vi "FeedbackDecode_20200902.vi"() -> ()   [LabVIEW 2016] (continued)
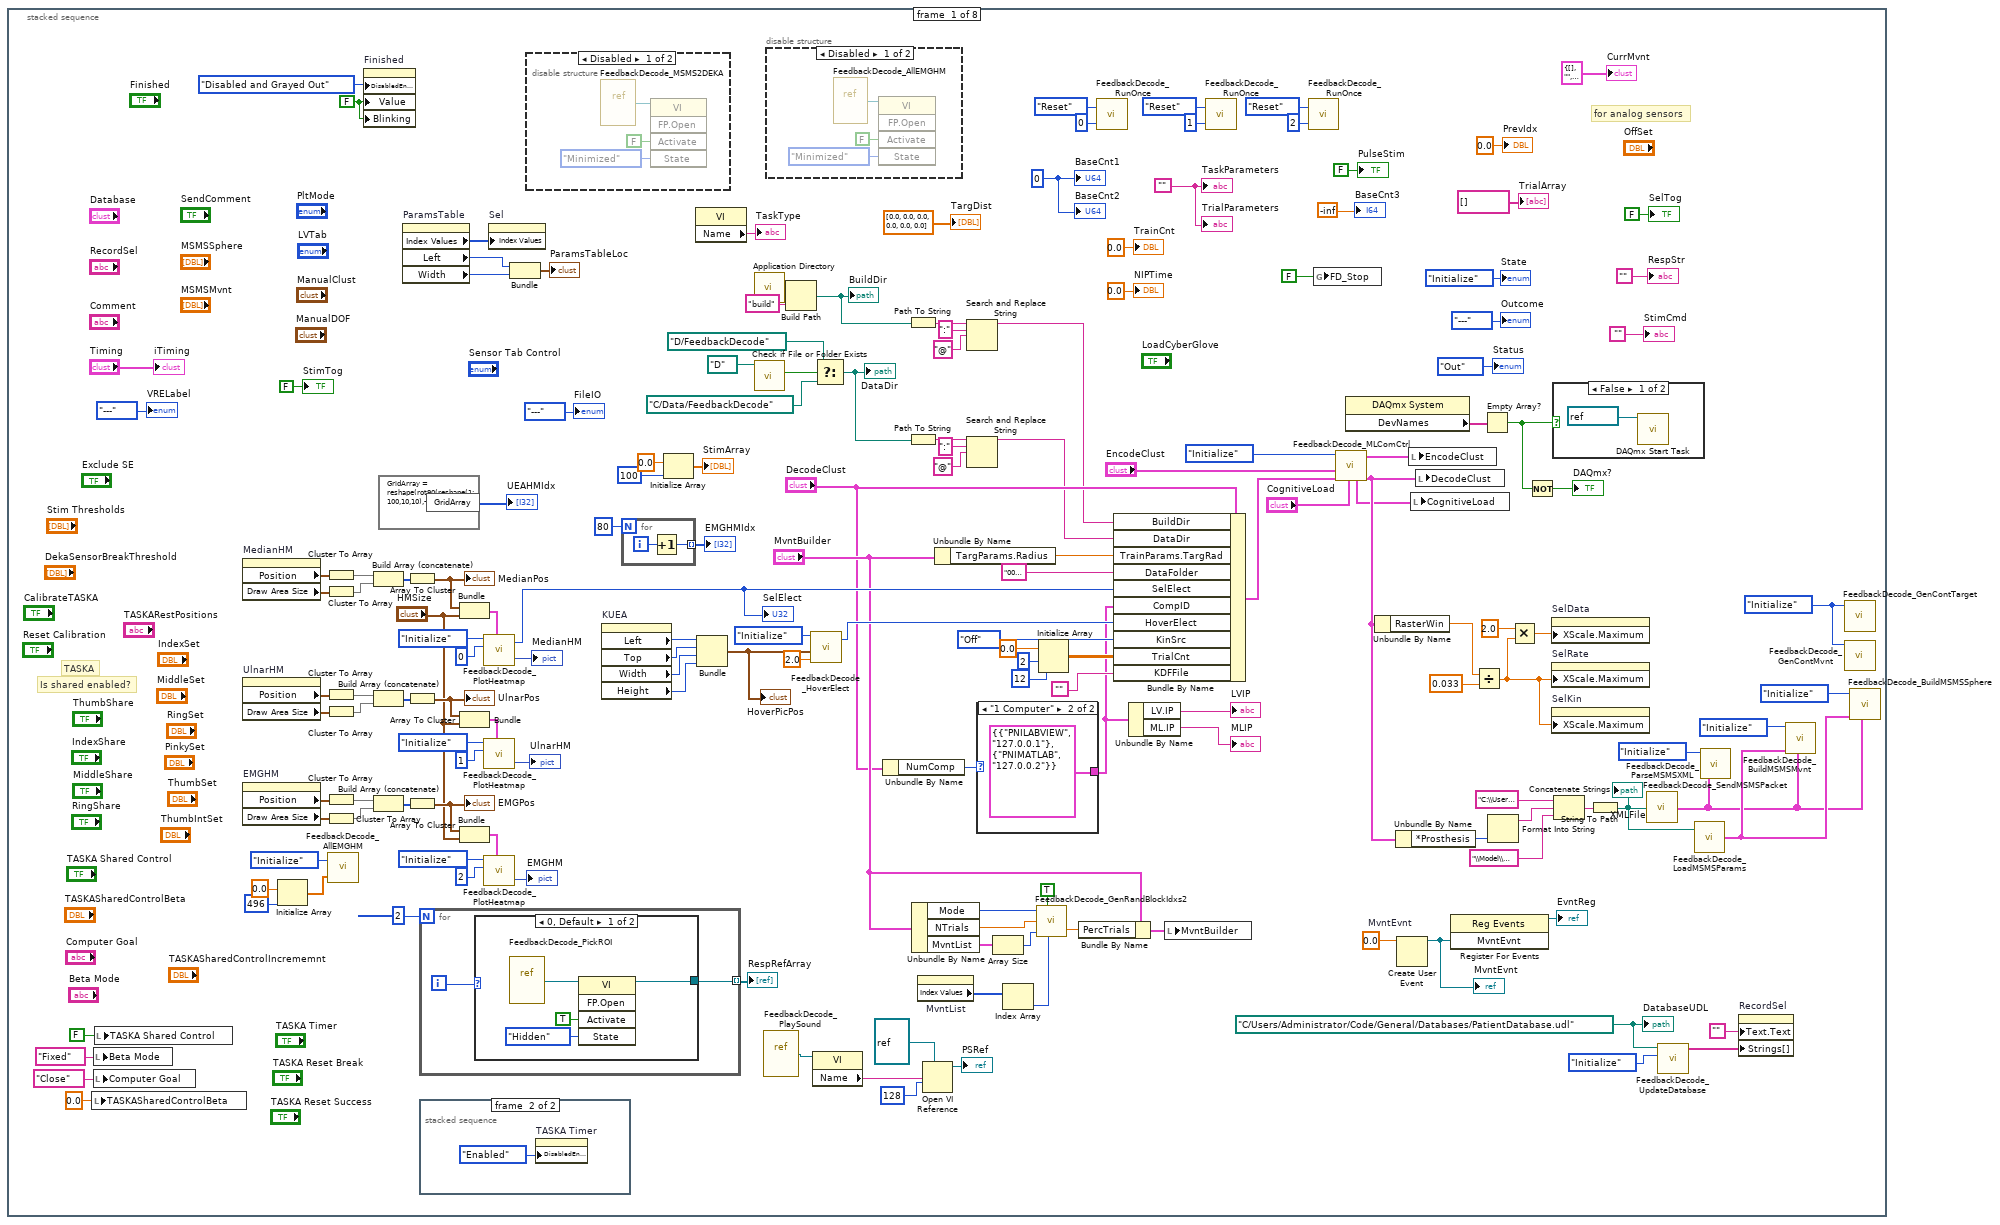
[diagram p2: hidden frame]
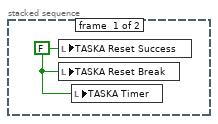
[diagram p3: hidden frame]
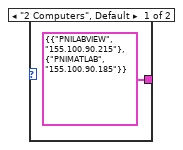
[diagram p4: hidden frame]
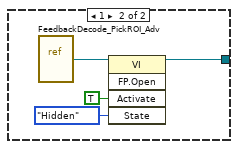
[diagram p7: hidden frame]
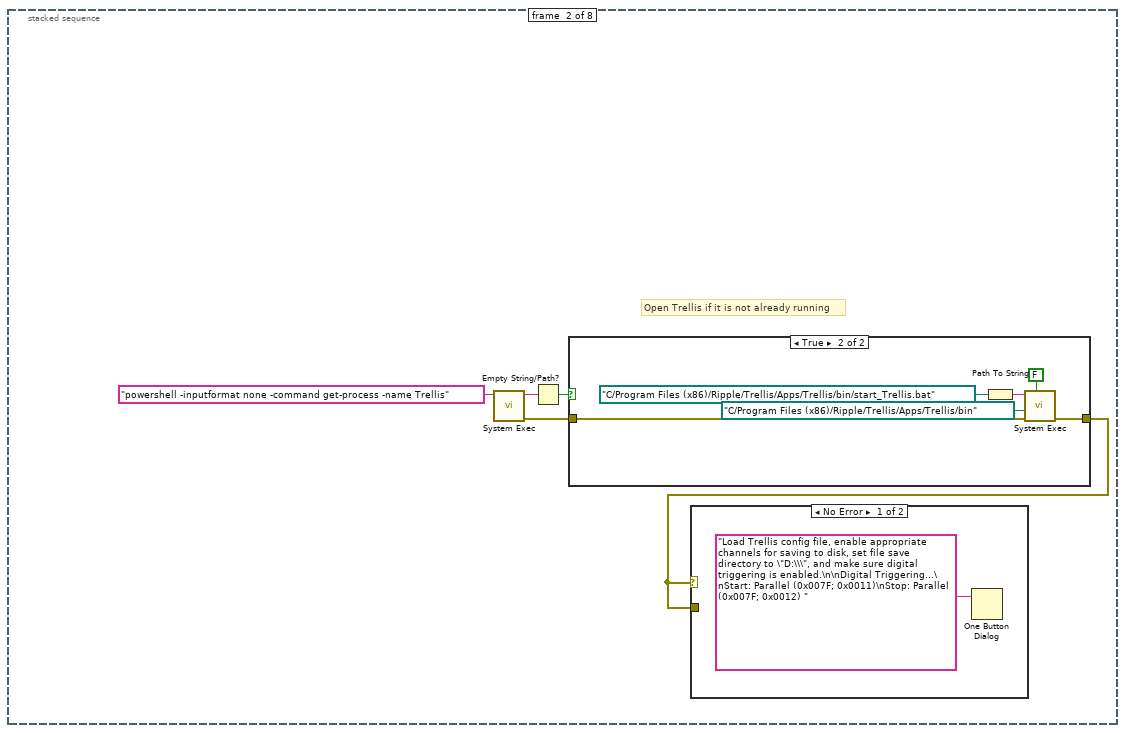
[diagram p9: hidden frame]
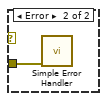
[diagram p11: hidden frame]
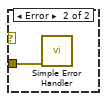
[diagram p14: hidden frame]
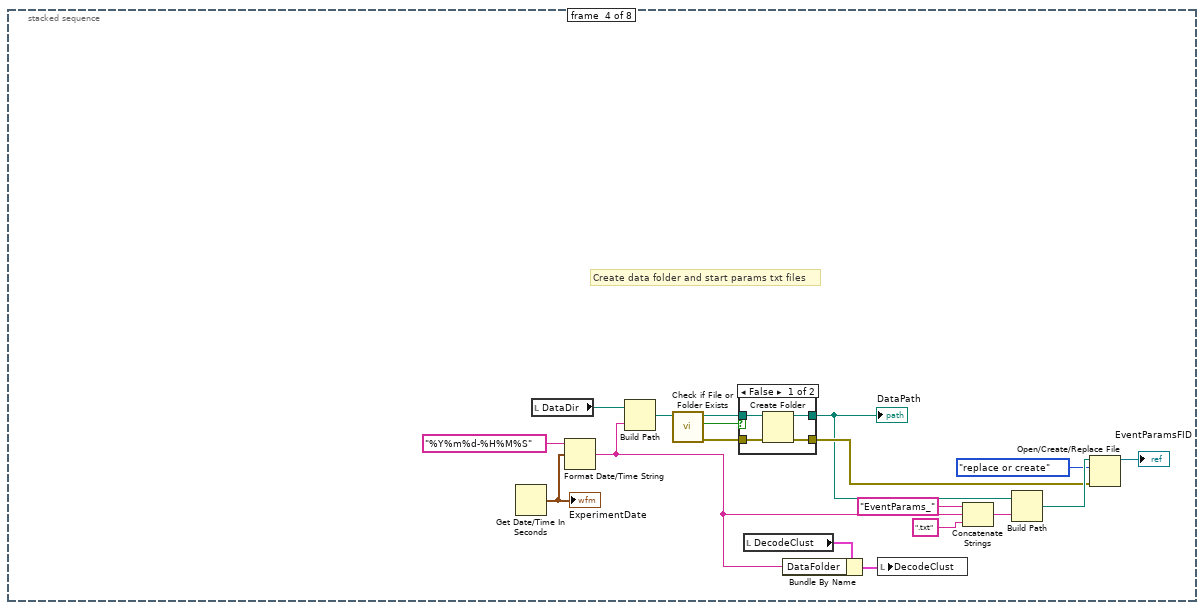
[diagram p15: hidden frame]
              }
              frame False {
                n2368 = property on="TASKA Timer" class="Bool (strict)"("DisabledEnum"=T17."Disabled and Grayed Out" ("Disabled")) -> ()  [unwired: 2 in, 2 out]
                n2369 = local read "LoopCnt"() -> (w2592:u64)
                n2370 = local read "NIPTime"() -> (w2595:dbl)
                n2371 = Format Into String(w2592) -> (resulting string=w2599:string)  [unwired: 3 in, 1 out]
                n2372 = local read "EventParamsFID"() -> (w2589:refnum<file>)
                n2373 = Concatenate Strings("SharedControlStopTime:SS.EventID=" ("string"), w2599) -> (w2593:string)
                n2374 = call-poly "FeedbackDecode_VariablesToString.vi"("Format"="%0.0f", "ValueIn"=w2595, "FieldName"="NIPTime" ("Key Word")) -> ("StringOut"=w2598:string)  [unwired: 4 in]
                n2375 = Concatenate Strings(w2593, ";", w2598) -> (w2594:string)
                n2376 = call "FeedbackDecode_WriteTextEOL.vi"("text"=w2594, "refnum in"=w2589) -> ()  [unwired: 8 in, 2 out]
              }
            }
          }
          event "TASKA Reset Break": Value Change {
            n2377 = event-data() -> ()  [unwired: 1 in, 6 out]
            n2378 = call-poly "FeedbackDecode_VariablesToString.vi"("Format"="%0.0f", "ValueIn"=0.0, "FieldName"="SharedControlTrialSuccess" ("Key Word")) -> ("StringOut"=w2601:string)  [unwired: 4 in]
            n2379 = property on="TASKA Timer" class="Bool (strict)"("DisabledEnum"=T17."Enabled" ("Disabled")) -> ()  [unwired: 2 in, 2 out]
            n2380 = local read "LoopCnt"() -> (w2608:u64)
            n2381 = local read "NIPTime"() -> (w2611:dbl)
            n2382 = Format Into String(w2608) -> (resulting string=w2615:string)  [unwired: 3 in, 1 out]
            n2383 = local read "EventParamsFID"() -> (w2605:refnum<file>)
            n2384 = Concatenate Strings("SharedControlTrialResult:SS.EventID=" ("string"), w2615) -> (w2609:string)
            n2385 = call-poly "FeedbackDecode_VariablesToString.vi"("Format"="%0.0f", "ValueIn"=w2611, "FieldName"="NIPTime" ("Key Word")) -> ("StringOut"=w2614:string)  [unwired: 4 in]
            n2386 = Concatenate Strings(w2609, ";", w2601, w2614) -> (w2610:string)
            n2387 = call "FeedbackDecode_WriteTextEOL.vi"("text"=w2610, "refnum in"=w2605) -> ()  [unwired: 8 in, 2 out]
          }
          event "TASKA Reset Success": Value Change {
            n2388 = event-data() -> ()  [unwired: 1 in, 6 out]
            n2389 = call-poly "FeedbackDecode_VariablesToString.vi"("Format"="%0.0f", "ValueIn"=1.0, "FieldName"="SharedControlTrialSuccess" ("Key Word")) -> ("StringOut"=w2618:string)  [unwired: 4 in]
            n2390 = property on="TASKA Timer" class="Bool (strict)"("DisabledEnum"=T17."Enabled" ("Disabled")) -> ()  [unwired: 2 in, 2 out]
            n2391 = local read "LoopCnt"() -> (w2625:u64)
            n2392 = local read "NIPTime"() -> (w2628:dbl)
            n2393 = Format Into String(w2625) -> (resulting string=w2632:string)  [unwired: 3 in, 1 out]
            n2394 = local read "EventParamsFID"() -> (w2622:refnum<file>)
            n2395 = Concatenate Strings("SharedControlTrialResult:SS.EventID=" ("string"), w2632) -> (w2626:string)
            n2396 = call-poly "FeedbackDecode_VariablesToString.vi"("Format"="%0.0f", "ValueIn"=w2628, "FieldName"="NIPTime" ("Key Word")) -> ("StringOut"=w2631:string)  [unwired: 4 in]
            n2397 = Concatenate Strings(w2626, ";", w2618, w2631) -> (w2627:string)
            n2398 = call "FeedbackDecode_WriteTextEOL.vi"("text"=w2627, "refnum in"=w2622) -> ()  [unwired: 8 in, 2 out]
          }
          event "TASKASharedControlBeta": Value Change {
            n2399 = event-data() -> ("NewVal"=w2634:dbl)  [unwired: 1 in, 5 out]
            n2400 = local read "LoopCnt"() -> (w2644:u64)
            n2401 = call-poly "FeedbackDecode_VariablesToString.vi"("Format"="%0.5f", "ValueIn"=w2634, "FieldName"="TASKASensors.SharedControl.Beta") -> ("StringOut"=w2651:string)  [unwired: 4 in]
            n2402 = local read "NIPTime"() -> (w2640:dbl)
            n2403 = Format Into String(w2644) -> (resulting string=w2636:string)  [unwired: 3 in, 1 out]
            n2404 = local read "EventParamsFID"() -> (w2648:refnum<file>)
            n2405 = local read "DecodeClust"() -> (w2649:T5)
            n2406 = Concatenate Strings("SharedControl:SS.EventID=" ("string"), w2636) -> (w2643:string)
            n2407 = call-poly "FeedbackDecode_VariablesToString.vi"("Format"="%0.0f", "ValueIn"=w2640, "FieldName"="NIPTime" ("Key Word")) -> ("StringOut"=w2637:string)  [unwired: 4 in]
            n2408 = Concatenate Strings(w2643, ";", w2651, w2637) -> (w2642:string)
            n2409 = call "FeedbackDecode_WriteTextEOL.vi"("text"=w2642, "refnum in"=w2648) -> ()  [unwired: 8 in, 2 out]
            n2410 = Bundle By Name(cluster=w2649, "EventStr"=w2642) -> (w2641:T5)
            n2411 = call "FeedbackDecode_MLComCtrl.vi"("DecodeClustIn"=w2641, "Mode"=T19."SendEvent") -> ()  [unwired: 6 in, 4 out]
          }
          event "TASKASharedControlIncrememnt": Value Change {
            n2412 = event-data() -> ("NewVal"=w2653:dbl)  [unwired: 1 in, 5 out]
            n2413 = local read "LoopCnt"() -> (w2663:u64)
            n2414 = call-poly "FeedbackDecode_VariablesToString.vi"("Format"="%0.5f", "ValueIn"=w2653, "FieldName"="TASKASensors.SharedControl.Increment") -> ("StringOut"=w2670:string)  [unwired: 4 in]
            n2415 = local read "NIPTime"() -> (w2659:dbl)
            n2416 = Format Into String(w2663) -> (resulting string=w2655:string)  [unwired: 3 in, 1 out]
            n2417 = local read "EventParamsFID"() -> (w2667:refnum<file>)
            n2418 = local read "DecodeClust"() -> (w2668:T5)
            n2419 = Concatenate Strings("SharedControl:SS.EventID=" ("string"), w2655) -> (w2662:string)
            n2420 = call-poly "FeedbackDecode_VariablesToString.vi"("Format"="%0.0f", "ValueIn"=w2659, "FieldName"="NIPTime" ("Key Word")) -> ("StringOut"=w2656:string)  [unwired: 4 in]
            n2421 = Concatenate Strings(w2662, ";", w2670, w2656) -> (w2661:string)
            n2422 = call "FeedbackDecode_WriteTextEOL.vi"("text"=w2661, "refnum in"=w2667) -> ()  [unwired: 8 in, 2 out]
            n2423 = Bundle By Name(cluster=w2668, "EventStr"=w2661) -> (w2660:T5)
            n2424 = call "FeedbackDecode_MLComCtrl.vi"("DecodeClustIn"=w2660, "Mode"=T19."SendEvent") -> ()  [unwired: 6 in, 4 out]
          }
          event "IndexSet", "MiddleSet", "RingSet", "PinkySet", "ThumbSet", "ThumbIntSet": Value Change {
            n2425 = event-data() -> ()  [unwired: 1 in, 6 out]
            n2426 = local read "ThumbIntSet"() -> (w2672:dbl)
            n2427 = local read "ThumbSet"() -> (w2673:dbl)
            n2428 = local read "MiddleSet"() -> (w2678:dbl)
            n2429 = local read "RingSet"() -> (w2677:dbl)
            n2430 = local read "PinkySet"() -> (w2674:dbl)
            n2431 = local read "IndexSet"() -> (w2679:dbl)
            n2432 = Build Array(w2679, w2678, w2677, w2674, w2673, w2672) -> (w2676:dbl[])
            n2433 = local read "LoopCnt"() -> (w2688:u64)
            n2434 = call-poly "FeedbackDecode_VariablesToString.vi"("Format"="%0.5f", "ValueIn"=w2676, "FieldName"="TASKA.RestPositions") -> ("StringOut"=w2695:string)  [unwired: 4 in]
            n2435 = local read "NIPTime"() -> (w2684:dbl)
            n2436 = Format Into String(w2688) -> (resulting string=w2681:string)  [unwired: 3 in, 1 out]
            n2437 = local read "EventParamsFID"() -> (w2692:refnum<file>)
            n2438 = local read "DecodeClust"() -> (w2693:T5)
            n2439 = Concatenate Strings("SharedControl:SS.EventID=" ("string"), w2681) -> (w2687:string)
            n2440 = call-poly "FeedbackDecode_VariablesToString.vi"("Format"="%0.0f", "ValueIn"=w2684, "FieldName"="NIPTime" ("Key Word")) -> ("StringOut"=w2675:string)  [unwired: 4 in]
            n2441 = Concatenate Strings(w2687, ";", w2695, w2675) -> (w2686:string)
            n2442 = call "FeedbackDecode_WriteTextEOL.vi"("text"=w2686, "refnum in"=w2692) -> ()  [unwired: 8 in, 2 out]
            n2443 = Bundle By Name(cluster=w2693, "EventStr"=w2686) -> (w2685:T5)
            n2444 = call "FeedbackDecode_MLComCtrl.vi"("DecodeClustIn"=w2685, "Mode"=T19."SendEvent") -> ()  [unwired: 6 in, 4 out]
          }
          event "ThumbShare", "IndexShare", "MiddleShare", "RingShare": Value Change {
            n2445 = event-data() -> ()  [unwired: 1 in, 6 out]
            n2446 = local read "ThumbShare"() -> (w2700:bool)
            n2447 = local read "MiddleShare"() -> (w2704:bool)
            n2448 = local read "RingShare"() -> (w2703:bool)
            n2449 = local read "IndexShare"() -> (w2705:bool)
            n2450 = Build Array(w2705, w2704, w2703, FALSE ("element"), w2700, FALSE ("element")) -> (w2698:bool[])
            n2451 = for {
              tunnel: w2698 -> [w2724] mode=indexing
              tunnel: [w2723] -> w2697 mode=indexing
              n2452 = case shown="False" w2724 {
                tunnel: [0.0 ("ValueIn") 1.0 ("ValueIn")] -> w2723
                frame False {
                }
                frame True {
                }
              }
            }
            n2453 = local read "LoopCnt"() -> (w2714:u64)
            n2454 = local read "NIPTime"() -> (w2710:dbl)
            n2455 = call-poly "FeedbackDecode_VariablesToString.vi"("Format"="%1.0f", "ValueIn"=w2697, "FieldName"="TASKASensors.SharedEnabled") -> ("StringOut"=w2721:string)  [unwired: 4 in]
            n2456 = Format Into String(w2714) -> (resulting string=w2707:string)  [unwired: 3 in, 1 out]
            n2457 = local read "EventParamsFID"() -> (w2718:refnum<file>)
            n2458 = local read "DecodeClust"() -> (w2719:T5)
            n2459 = Concatenate Strings("SharedControl:SS.EventID=" ("string"), w2707) -> (w2713:string)
            n2460 = call-poly "FeedbackDecode_VariablesToString.vi"("Format"="%0.0f", "ValueIn"=w2710, "FieldName"="NIPTime" ("Key Word")) -> ("StringOut"=w2702:string)  [unwired: 4 in]
            n2461 = Concatenate Strings(w2713, ";", w2721, w2702) -> (w2712:string)
            n2462 = call "FeedbackDecode_WriteTextEOL.vi"("text"=w2712, "refnum in"=w2718) -> ()  [unwired: 8 in, 2 out]
            n2463 = Bundle By Name(cluster=w2719, "EventStr"=w2712) -> (w2711:T5)
            n2464 = call "FeedbackDecode_MLComCtrl.vi"("DecodeClustIn"=w2711, "Mode"=T19."SendEvent") -> ()  [unwired: 6 in, 4 out]
          }
          event "Computer Goal": Value Change {
            n2465 = event-data() -> ("NewVal"=w2727:string)  [unwired: 1 in, 5 out]
            n2466 = local read "LoopCnt"() -> (w2737:u64)
            n2467 = call-poly "FeedbackDecode_VariablesToString.vi"("Format"="%0.5f", "ValueIn"=w2727, "FieldName"="TASKASensors.SharedControl.ComputerGoal") -> ("StringOut"=w2744:string)  [unwired: 4 in]
            n2468 = local read "NIPTime"() -> (w2733:dbl)
            n2469 = Format Into String(w2737) -> (resulting string=w2729:string)  [unwired: 3 in, 1 out]
            n2470 = local read "EventParamsFID"() -> (w2741:refnum<file>)
            n2471 = local read "DecodeClust"() -> (w2742:T5)
            n2472 = Concatenate Strings("SharedControl:SS.EventID=" ("string"), w2729) -> (w2736:string)
            n2473 = call-poly "FeedbackDecode_VariablesToString.vi"("Format"="%0.0f", "ValueIn"=w2733, "FieldName"="NIPTime" ("Key Word")) -> ("StringOut"=w2730:string)  [unwired: 4 in]
            n2474 = Concatenate Strings(w2736, ";", w2744, w2730) -> (w2735:string)
            n2475 = call "FeedbackDecode_WriteTextEOL.vi"("text"=w2735, "refnum in"=w2741) -> ()  [unwired: 8 in, 2 out]
            n2476 = Bundle By Name(cluster=w2742, "EventStr"=w2735) -> (w2734:T5)
            n2477 = call "FeedbackDecode_MLComCtrl.vi"("DecodeClustIn"=w2734, "Mode"=T19."SendEvent") -> ()  [unwired: 6 in, 4 out]
          }
          event "Beta Mode": Value Change {
            n2478 = event-data() -> ("NewVal"=w2746:string)  [unwired: 1 in, 5 out]
            n2479 = local read "LoopCnt"() -> (w2756:u64)
            n2480 = call-poly "FeedbackDecode_VariablesToString.vi"("Format"="%0.5f", "ValueIn"=w2746, "FieldName"="TASKASensors.SharedControl.BetaMode") -> ("StringOut"=w2763:string)  [unwired: 4 in]
            n2481 = local read "NIPTime"() -> (w2752:dbl)
            n2482 = Format Into String(w2756) -> (resulting string=w2748:string)  [unwired: 3 in, 1 out]
            n2483 = local read "EventParamsFID"() -> (w2760:refnum<file>)
            n2484 = local read "DecodeClust"() -> (w2761:T5)
            n2485 = Concatenate Strings("SharedControl:SS.EventID=" ("string"), w2748) -> (w2755:string)
            n2486 = call-poly "FeedbackDecode_VariablesToString.vi"("Format"="%0.0f", "ValueIn"=w2752, "FieldName"="NIPTime" ("Key Word")) -> ("StringOut"=w2749:string)  [unwired: 4 in]
            n2487 = Concatenate Strings(w2755, ";", w2763, w2749) -> (w2754:string)
            n2488 = call "FeedbackDecode_WriteTextEOL.vi"("text"=w2754, "refnum in"=w2760) -> ()  [unwired: 8 in, 2 out]
            n2489 = Bundle By Name(cluster=w2761, "EventStr"=w2754) -> (w2753:T5)
            n2490 = call "FeedbackDecode_MLComCtrl.vi"("DecodeClustIn"=w2753, "Mode"=T19."SendEvent") -> ()  [unwired: 6 in, 4 out]
          }
          event Mouse Wheel; Mouse Down; Mouse Move {
            n2491 = event-data() -> ("CtlRef"=w2765:refnum<vi>)  [unwired: 1 in, 4 out]
            n2492 = property class="Arr (strict)"(reference=w2765) -> ("Index Values"=w2766:u32[])  [unwired: 1 in, 2 out]
            n2493 = Index Array(array=w2766) -> (element=w2767:u32)  [unwired: 1 in]
            n2494 = Build Array(w2767) -> (w2768:u32[])
            n2495 = property on="Sel" class="Arr (strict)"("Index Values"=w2768) -> ()  [unwired: 2 in, 2 out]
          }
          event "RespStr": Value Change {
            n2496 = event-data() -> ("NewVal"=w2770:string)  [unwired: 1 in, 5 out]
            n2497 = Empty String/Path?(string/path=w2770) -> (empty?=w2771:bool)
            n2498 = case shown="False" w2771 {
              tunnel: w2770 -> [w2775 _]
              frame False {
                n2499 = xnode "Match Regular Expression"("input string"=w2775, "regular expression"="Sensor='") -> ("after match"=w2778:string)  [unwired: 4 in, 4 out]
                n2500 = local read "EncodeClust"() -> (w2780:T9)
                n2501 = xnode "Match Regular Expression"("input string"=w2778, "regular expression"="';") -> ("before match"=w2774:string)  [unwired: 4 in, 4 out]
                n2502 = call "FeedbackDecode_UpdateRegion.vi"("EncodeClustIn"=w2780, "RegionStr"=w2774) -> ("EncodeClustOut"=w2779:T9)  [unwired: 1 in]
                n2503 = local write "EncodeClust"(w2779) -> ()
                n2504 = local read "LoopCnt"() -> (w2790:u64)
                n2505 = local read "NIPTime"() -> (w2786:dbl)
                n2506 = local read "StimCmd"() -> (w2773:string)
                n2507 = Format Into String(w2790) -> (resulting string=w2781:string)  [unwired: 3 in, 1 out]
                n2508 = call-poly "FeedbackDecode_VariablesToString.vi"("Format"="%0.0f", "ValueIn"=w2786, "FieldName"="NIPTime" ("Key Word")) -> ("StringOut"=w2783:string)  [unwired: 4 in]
                n2509 = Concatenate Strings("Response:SS.EventID=" ("string"), w2781) -> (w2789:string)
                n2510 = local read "EventParamsFID"() -> (w2793:refnum<file>)
                n2511 = Concatenate Strings(w2789, ";", w2775, w2773, w2783) -> (w2788:string)
                n2512 = local read "DecodeClust"() -> (w2794:T5)
                n2513 = call "FeedbackDecode_WriteTextEOL.vi"("text"=w2788, "refnum in"=w2793) -> ()  [unwired: 8 in, 2 out]
                n2514 = Bundle By Name(cluster=w2794, "EventStr"=w2788) -> (w2787:T5)
                n2515 = call "FeedbackDecode_MLComCtrl.vi"("DecodeClustIn"=w2787, "Mode"=T19."SendEvent") -> ()  [unwired: 6 in, 4 out]
              }
              frame True {
              }
            }
          }
          event Value Change {
            n2516 = event-data() -> ("NewVal"=w3023:bool)  [unwired: 1 in, 5 out]
            n2517 = case shown="True" w3023 {
              frame False {
              }
              frame True {
                n2518 = local read "EncodeClust"() -> (w3027:T9)
                n2519 = Bundle By Name(cluster=w3027, "RespClust.OpenResp"=FALSE ("OpenResp")) -> (w3029:T9)
                n2520 = local read "RespRefArray"() -> (w3028:refnum<vi>[])
                n2521 = local write "EncodeClust"(w3029) -> ()
                n2522 = Unbundle By Name(w3027) -> ("RespClust.RespType"=w3026:enum16{"Sensor Map", "Full Map"})
                n2523 = Index Array(array=w3028, index=w3026) -> (element=w3025:refnum<vi>)
                n2524 = invoke class="VI" method="FP.Open"(reference=w3025, "Activate"=TRUE ("Activate?"), "State"=T21."Standard") -> (reference out=w3034:refnum<vi>)  [unwired: 2 in, 4 out]
                n2525 = property class="VI"(reference=w3034, "Front Panel.IsFrontmost"=TRUE ("Front Panel Window:Is Frontmost")) -> ()  [unwired: 1 in, 2 out]
                n2526 = local read "LoopCnt"() -> (w3044:u64)
                n2527 = local read "NIPTime"() -> (w3040:dbl)
                n2528 = Format Into String(w3044) -> (resulting string=w3035:string)  [unwired: 3 in, 1 out]
                n2529 = call-poly "FeedbackDecode_VariablesToString.vi"("Format"="%0.0f", "ValueIn"=w3040, "FieldName"="NIPTime" ("Key Word")) -> ("StringOut"=w3037:string)  [unwired: 4 in]
                n2530 = Concatenate Strings("OpenResp:SS.EventID=" ("string"), w3035) -> (w3043:string)
                n2531 = local read "EventParamsFID"() -> (w3047:refnum<file>)
                n2532 = Concatenate Strings(w3043, ";", w3037) -> (w3042:string)
                n2533 = local read "DecodeClust"() -> (w3048:T5)
                n2534 = call "FeedbackDecode_WriteTextEOL.vi"("text"=w3042, "refnum in"=w3047) -> ()  [unwired: 8 in, 2 out]
                n2535 = Bundle By Name(cluster=w3048, "EventStr"=w3042) -> (w3041:T5)
                n2536 = call "FeedbackDecode_MLComCtrl.vi"("DecodeClustIn"=w3041, "Mode"=T19."SendEvent") -> ()  [unwired: 6 in, 4 out]
              }
            }
          }
          event Value Change {
            n2537 = event-data() -> ("NewVal"=w3073:T52)  [unwired: 1 in, 5 out]
            n2538 = Cluster To Array(cluster=w3073) -> (array=w3072:bool[])
            n2539 = Search 1D Array(1D array=w3072, element=TRUE) -> (index of element=w3049:i32)  [unwired: 1 in]
            n2540 = local read "EncodeClust"() -> (w3050:T9)
            n2541 = call "FeedbackDecode_SortParamsTable.vi"("StimClustIn"=w3050, "Column"=w3049) -> ("StimClustOut"=w3070:T9)  [unwired: 1 in]
            n2542 = call "FeedbackDecode_Params2Preset.vi"("StimClustIn"=w3070) -> ("StimClustOut"=w3069:T9)  [unwired: 2 in]
            n2543 = local read "LoopCnt"() -> (w3061:u64)
            n2544 = call "FeedbackDecode_UpdateParamsTable.vi"("StimClustIn"=w3069) -> ("StimClustOut"=w3068:T9)  [unwired: 2 in]
            n2545 = call "FeedbackDecode_Params2UEA.vi"("StimClustIn"=w3068) -> ("StimClustOut"=w3067:T9)  [unwired: 2 in]
            n2546 = Format Into String(w3061) -> (resulting string=w3053:string)  [unwired: 3 in, 1 out]
            n2547 = local read "NIPTime"() -> (w3057:dbl)
            n2548 = call "FeedbackDecode_BuildStimCmd.vi"("EncodeClustIn"=w3067) -> ("EncodeClustOut"=w3052:T9, "StimCmd"=w3051:string)  [unwired: 1 in]
            n2549 = local read "EventParamsFID"() -> (w3065:refnum<file>)
            n2550 = Concatenate Strings("SortStim:SS.EventID=" ("string"), w3053) -> (w3060:string)
            n2551 = call-poly "FeedbackDecode_VariablesToString.vi"("Format"="%0.0f", "ValueIn"=w3057, "FieldName"="NIPTime" ("Key Word")) -> ("StringOut"=w3054:string)  [unwired: 4 in]
            n2552 = local read "DecodeClust"() -> (w3066:T5)
            n2553 = Concatenate Strings(w3060, ";", w3051, w3054) -> (w3059:string)
            n2554 = call "FeedbackDecode_WriteTextEOL.vi"("text"=w3059, "refnum in"=w3065) -> ()  [unwired: 8 in, 2 out]
            n2555 = Bundle By Name(cluster=w3066, "EventStr"=w3059) -> (w3058:T5)
            n2556 = local write "StimCmd"(w3051) -> ()
            n2557 = local write "EncodeClust"(w3052) -> ()
            n2558 = call "FeedbackDecode_MLComCtrl.vi"("DecodeClustIn"=w3058, "Mode"=T19."SendEvent") -> ()  [unwired: 6 in, 4 out]
          }
          event Value Change {
            n2559 = event-data() -> ()  [unwired: 1 in, 6 out]
            n2560 = local read "EncodeClust"() -> (w3076:T9)
            n2561 = Unbundle By Name(w3076) -> ("Sel"=w3077:bool[])
            n2562 = local read "SelTog"() -> (w3080:bool)
            n2563 = case shown="False" w3080 {
              selector: w3080 -> [w3102 w3108]
              tunnel: w3077 -> [w3106 w3112]
              tunnel: [w3103 w3109] -> w3078
              frame True {
                n2564 = Not(x=w3102) -> (.not. x?=w3101:bool)
                n2565 = Array Size(array=w3106) -> (size(s)=w3105:i32)
                n2566 = local write "SelTog"(w3101) -> ()
                n2567 = Initialize Array(FALSE, w3105) -> (w3103:bool[])
              }
              frame False {
                n2568 = Not(x=w3108) -> (.not. x?=w3107:bool)
                n2569 = Array Size(array=w3112) -> (size(s)=w3111:i32)
                n2570 = local write "SelTog"(w3107) -> ()
                n2571 = Initialize Array(TRUE, w3111) -> (w3109:bool[])
              }
            }
            n2572 = Bundle By Name(cluster=w3076, "Sel"=w3078, "SelSort.Sel"=FALSE) -> (w3075:T9)
            n2573 = call "FeedbackDecode_Params2Preset.vi"("StimClustIn"=w3075) -> ("StimClustOut"=w3099:T9)  [unwired: 2 in]
            n2574 = local read "LoopCnt"() -> (w3091:u64)
            n2575 = call "FeedbackDecode_UpdateParamsTable.vi"("StimClustIn"=w3099) -> ("StimClustOut"=w3098:T9)  [unwired: 2 in]
            n2576 = call "FeedbackDecode_Params2UEA.vi"("StimClustIn"=w3098) -> ("StimClustOut"=w3097:T9)  [unwired: 2 in]
            n2577 = Format Into String(w3091) -> (resulting string=w3083:string)  [unwired: 3 in, 1 out]
            n2578 = local read "NIPTime"() -> (w3087:dbl)
            n2579 = call "FeedbackDecode_BuildStimCmd.vi"("EncodeClustIn"=w3097) -> ("EncodeClustOut"=w3082:T9, "StimCmd"=w3081:string)  [unwired: 1 in]
            n2580 = local read "EventParamsFID"() -> (w3095:refnum<file>)
            n2581 = Concatenate Strings("SortStim:SS.EventID=" ("string"), w3083) -> (w3090:string)
            n2582 = call-poly "FeedbackDecode_VariablesToString.vi"("Format"="%0.0f", "ValueIn"=w3087, "FieldName"="NIPTime" ("Key Word")) -> ("StringOut"=w3084:string)  [unwired: 4 in]
            n2583 = local read "DecodeClust"() -> (w3096:T5)
            n2584 = Concatenate Strings(w3090, ";", w3081, w3084) -> (w3089:string)
            n2585 = call "FeedbackDecode_WriteTextEOL.vi"("text"=w3089, "refnum in"=w3095) -> ()  [unwired: 8 in, 2 out]
            n2586 = Bundle By Name(cluster=w3096, "EventStr"=w3089) -> (w3088:T5)
            n2587 = local write "StimCmd"(w3081) -> ()
            n2588 = local write "EncodeClust"(w3082) -> ()
            n2589 = call "FeedbackDecode_MLComCtrl.vi"("DecodeClustIn"=w3088, "Mode"=T19."SendEvent") -> ()  [unwired: 6 in, 4 out]
          }
          event Key Down {
            n2590 = event-data() -> ("Char"=w3114:i16, "VKey"=w3115:T53)  [unwired: 1 in, 8 out]
            n2591 = local read "LVTab"() -> (w3113:T4)
            n2592 = case shown="\"Encode\"" w3113 {
              tunnel: w3115 -> [_ w3118]
              tunnel: w3114 -> [_ w3117]
              frame "Decode", Default {
              }
              frame "Encode" {
                n2593 = case shown="\"Up\"" w3118 {
                  tunnel: w3117 -> [w3119 _ _ _ _ _]
                  frame "ASCII" {
                    n2594 = case shown="115" w3119 {
                      frame -1, Default {
                      }
                      frame 115 {
                        # "s=stim"
                        n2595 = disable-structure shown="Disabled" {
                          frame Disabled {
                            n2596 = local read "StimTog"() -> (w3120:bool)
                            n2597 = case shown="True" w3120 {
                              selector: w3120 -> [w3122 w3124]
                              frame True {
                                n2598 = Not(x=w3122) -> (.not. x?=w3121:bool)
                                n2599 = local write "StimTog"(w3121) -> ()
                                n2600 = property on="Stim" class="Bool (strict)"("Val(Sgnl)"=w3121) -> ()  [unwired: 2 in, 2 out]
                              }
                              frame False {
                                n2601 = Not(x=w3124) -> (.not. x?=w3123:bool)
                                n2602 = local write "StimTog"(w3123) -> ()
                                n2603 = property on="Stim" class="Bool (strict)"("Val(Sgnl)"=w3123) -> ()  [unwired: 2 in, 2 out]
                              }
                            }
                          }
                          frame Enabled {
                          }
                        }
                      }
                    }
                  }
                  frame Default {
                  }
                  frame "Up" {
                    n2604 = property on="Add" class="Bool (strict)"("Val(Sgnl)"=TRUE ("Value (Signaling)")) -> ()  [unwired: 2 in, 2 out]
                  }
                  frame "Down" {
                    n2605 = property on="Sub" class="Bool (strict)"("Val(Sgnl)"=TRUE ("Value (Signaling)")) -> ()  [unwired: 2 in, 2 out]
                  }
                  frame "Left" {
                    w3132 = 100 ("length")
                    n2606 = local read "EncodeClust"() -> (w3145:T9)
                    n2607 = Unbundle By Name(w3145) -> ("UEAArray"=w3140:T25)
                    n2608 = Index Array(array=w3140) -> (element #1=w3141:T54, element #2=w3142:T54)  [unwired: 2 in]
                    n2609 = Cluster To Array(cluster=w3141) -> (array=w3143:bool[])
                    n2610 = Cluster To Array(cluster=w3142) -> (array=w3144:bool[])
                    n2611 = Build Array (concatenate)(w3143, w3144) -> (w3139:bool[])
                    n2612 = Search 1D Array(1D array=w3139, element=TRUE) -> (index of element=w3136:i32)  [unwired: 1 in]
                    n2613 = Decrement(x=w3136) -> (x-1=w3135:i32)
                    n2614 = Replace Array Subset(array=bool[] [FALSE, FALSE, FALSE, FALSE, FALSE, FALSE, FALSE, FALSE, FALSE, FALSE, FALSE, FALSE, FALSE, FALSE, FALSE, FALSE, FALSE, FALSE, FALSE, FALSE, FALSE, FALSE, FALSE, FALSE, FALSE, FALSE, FALSE, FALSE, FALSE, FALSE, FALSE, FALSE, FALSE, FALSE, FALSE, FALSE, FALSE, FALSE, FALSE, FALSE, FALSE, FALSE, FALSE, FALSE, FALSE, FALSE, FALSE, FALSE, FALSE, FALSE, FALSE, FALSE, FALSE, FALSE, FALSE, FALSE, FALSE, FALSE, FALSE, FALSE, FALSE, FALSE, FALSE, FALSE, FALSE, FALSE, FALSE, FALSE, FALSE, FALSE, FALSE, FALSE, FALSE, FALSE, FALSE, FALSE, FALSE, FALSE, FALSE, FALSE, FALSE, FALSE, FALSE, FALSE, FALSE, FALSE, FALSE, FALSE, FALSE, FALSE, FALSE, FALSE, FALSE, FALSE, FALSE, FALSE, FALSE, FALSE, FALSE, FALSE, FALSE, FALSE, FALSE, FALSE, FALSE, FALSE, FALSE, FALSE, FALSE, FALSE, FALSE, FALSE, FALSE, FALSE, FALSE, FALSE, FALSE, FALSE, FALSE, FALSE, FALSE, FALSE, FALSE, FALSE, FALSE, FALSE, FALSE, FALSE, FALSE, FALSE, FALSE, FALSE, FALSE, FALSE, FALSE, FALSE, FALSE, FALSE, FALSE, FALSE, FALSE, FALSE, FALSE, FALSE, FALSE, FALSE, FALSE, FALSE, FALSE, FALSE, FALSE, FALSE, FALSE, FALSE, FALSE, FALSE, FALSE, FALSE, FALSE, FALSE, FALSE, FALSE, FALSE, FALSE, FALSE, FALSE, FALSE, FALSE, FALSE, FALSE, FALSE, FALSE, FALSE, FALSE, FALSE, FALSE, FALSE, FALSE, FALSE, FALSE, FALSE, FALSE, FALSE, FALSE, FALSE, FALSE, FALSE, FALSE, FALSE, FALSE, FALSE, FALSE, FALSE, FALSE, FALSE, FALSE, FALSE, FALSE, FALSE, FALSE] ("appended array"), new element=TRUE, index=w3135) -> (w3133:bool[])
                    n2615 = Array Subset(array=w3133, length=w3132) -> (w3131:bool[])  [unwired: 1 in]
                    n2616 = Array Subset(array=w3133, index=w3132, length=w3132) -> (w3130:bool[])
                    n2617 = Array To Cluster(array=w3131) -> (cluster=w3129:T48)
                    n2618 = Array To Cluster(array=w3130) -> (cluster=w3128:T48)
                    n2619 = Build Array(w3129, w3128) -> (w3127:T55)
                    n2620 = property on="UEAArray" class="Arr (strict)"("Val(Sgnl)"=w3127) -> ()  [unwired: 2 in, 2 out]
                  }
                  frame "Right" {
                    w3151 = 100 ("length")
                    n2621 = local read "EncodeClust"() -> (w3164:T9)
                    n2622 = Unbundle By Name(w3164) -> ("UEAArray"=w3159:T25)
                    n2623 = Index Array(array=w3159) -> (element #1=w3160:T54, element #2=w3161:T54)  [unwired: 2 in]
                    n2624 = Cluster To Array(cluster=w3160) -> (array=w3162:bool[])
                    n2625 = Cluster To Array(cluster=w3161) -> (array=w3163:bool[])
                    n2626 = Build Array (concatenate)(w3162, w3163) -> (w3158:bool[])
                    n2627 = Search 1D Array(1D array=w3158, element=TRUE) -> (index of element=w3155:i32)  [unwired: 1 in]
                    n2628 = Increment(x=w3155) -> (x+1=w3154:i32)
                    n2629 = Replace Array Subset(array=bool[] [FALSE, FALSE, FALSE, FALSE, FALSE, FALSE, FALSE, FALSE, FALSE, FALSE, FALSE, FALSE, FALSE, FALSE, FALSE, FALSE, FALSE, FALSE, FALSE, FALSE, FALSE, FALSE, FALSE, FALSE, FALSE, FALSE, FALSE, FALSE, FALSE, FALSE, FALSE, FALSE, FALSE, FALSE, FALSE, FALSE, FALSE, FALSE, FALSE, FALSE, FALSE, FALSE, FALSE, FALSE, FALSE, FALSE, FALSE, FALSE, FALSE, FALSE, FALSE, FALSE, FALSE, FALSE, FALSE, FALSE, FALSE, FALSE, FALSE, FALSE, FALSE, FALSE, FALSE, FALSE, FALSE, FALSE, FALSE, FALSE, FALSE, FALSE, FALSE, FALSE, FALSE, FALSE, FALSE, FALSE, FALSE, FALSE, FALSE, FALSE, FALSE, FALSE, FALSE, FALSE, FALSE, FALSE, FALSE, FALSE, FALSE, FALSE, FALSE, FALSE, FALSE, FALSE, FALSE, FALSE, FALSE, FALSE, FALSE, FALSE, FALSE, FALSE, FALSE, FALSE, FALSE, FALSE, FALSE, FALSE, FALSE, FALSE, FALSE, FALSE, FALSE, FALSE, FALSE, FALSE, FALSE, FALSE, FALSE, FALSE, FALSE, FALSE, FALSE, FALSE, FALSE, FALSE, FALSE, FALSE, FALSE, FALSE, FALSE, FALSE, FALSE, FALSE, FALSE, FALSE, FALSE, FALSE, FALSE, FALSE, FALSE, FALSE, FALSE, FALSE, FALSE, FALSE, FALSE, FALSE, FALSE, FALSE, FALSE, FALSE, FALSE, FALSE, FALSE, FALSE, FALSE, FALSE, FALSE, FALSE, FALSE, FALSE, FALSE, FALSE, FALSE, FALSE, FALSE, FALSE, FALSE, FALSE, FALSE, FALSE, FALSE, FALSE, FALSE, FALSE, FALSE, FALSE, FALSE, FALSE, FALSE, FALSE, FALSE, FALSE, FALSE, FALSE, FALSE, FALSE, FALSE, FALSE, FALSE, FALSE, FALSE, FALSE, FALSE, FALSE, FALSE, FALSE, FALSE, FALSE] ("appended array"), new element=TRUE, index=w3154) -> (w3152:bool[])
                    n2630 = Array Subset(array=w3152, length=w3151) -> (w3150:bool[])  [unwired: 1 in]
                    n2631 = Array Subset(array=w3152, index=w3151, length=w3151) -> (w3149:bool[])
                    n2632 = Array To Cluster(array=w3150) -> (cluster=w3148:T48)
                    n2633 = Array To Cluster(array=w3149) -> (cluster=w3147:T48)
                    n2634 = Build Array(w3148, w3147) -> (w3146:T55)
                    n2635 = property on="UEAArray" class="Arr (strict)"("Val(Sgnl)"=w3146) -> ()  [unwired: 2 in, 2 out]
                  }
                }
              }
            }
          }
          event "ManualClust": Mouse Down {
            n2636 = event-data() -> ("Mods"=w3167:cluster{"Double Click":bool, "Menu Key":bool})  [unwired: 1 in, 7 out]
            n2637 = Unbundle By Name(w3167) -> ("Double Click"=w3165:bool)
            n2638 = case shown="True" w3165 {
              frame False {
              }
              frame True {
                n2639 = local write "ManualClust"(T7 {"Thumb"=0.0, "Index"=0.0, "Middle"=0.0, "Ring"=0.0, "Little"=0.0, "ThumbInt"=0.0, "IndexInt"=0.0, "RingInt"=0.0, "LittleInt"=0.0, "WristPitch"=0.0, "WristYaw"=0.0, "WristRoll"=0.0} ("ManualClust")) -> ()
              }
            }
          }
        }
      }
      n2640 = node-c288(w327) -> ()  [unwired: 1 out]
    }
    frame #2 {
      n2641 = stacked-sequence {
        frame #0 {
          # "Writing initial trial parameters to txt file and NIP"
          # "need to add an entry to TrialArray in case program finishes without running a trial (see RippleEMG)"
          n2642 = local read "MvntBuilder"() -> (w3802:T6)
          n2643 = local read "Timing"() -> (w3804:T3)
          n2644 = local read "CurrMvnt"() -> (w3801:T1)
          n2645 = Unbundle By Name(w3802) -> ("TargParams"=w3803:cluster{"Gain":dbl, "Radius":dbl, "Acc":dbl})
          n2646 = local read "DecodeClust"() -> (w3807:T5)
          n2647 = local read "TrialArray"() -> (w3805:string[])
          n2648 = local read "NIPTime"() -> (w3799:dbl)
          n2649 = call "FeedbackDecode_FPPNS2NIP.vi"("NIPTime"=w3799, "LoopCnt"=-1, "DecodeClust"=w3807, "TrialTiming"=w3804, "TargParams"=w3803, "MvntClust"=w3801) -> ("TrialParams"=w3806:string)  [unwired: 5 in]
          n2650 = local read "EventParamsFID"() -> (w3800:refnum<file>)
          n2651 = Insert Into Array(array=w3805, new element=w3806) -> (w3808:string[])  [unwired: 1 in]
          n2652 = local write "TrialArray"(w3808) -> ()
          n2653 = call "FeedbackDecode_WriteTextEOL.vi"("text"=w3806, "refnum in"=w3800) -> ()  [unwired: 8 in, 2 out]
        }
        frame #1 {
          w3812 = "_" ("string")
          w3814 = ".txt" ("string")
          # "Save Params and Preset Tables"
          n2654 = local read "DecodeClust"() -> (w3811:T5)
          n2655 = Unbundle By Name(w3811) -> ("DataFolder"=w3810:string)
          n2656 = Get Date/Time In Seconds() -> (seconds since 1Jan1904=w3823:timestamp)
          n2657 = Format Date/Time String(time format string (%c)="%H%M%S", seconds (now)=w3823) -> (date/time string=w3815:string)  [unwired: 1 in]
          n2658 = local read "EncodeClust"() -> (w3816:T9)
          n2659 = local read "DataPath"() -> (w3813:path)
          n2660 = Concatenate Strings("StimParams_" ("name or relative path"), w3810, w3812, w3815, w3814) -> (w3821:string)
          n2661 = Unbundle By Name(w3816) -> ("ParamsTable"=w3825:string[][])
          n2662 = Build Path(base path=w3813, name or relative path=w3821) -> (appended path=w3820:path)
          n2663 = Unbundle By Name(w3816) -> ("PresetTable"=w3809:string[][])
          n2664 = call-poly <vilib>:"Write Delimited Spreadsheet.vi"("file path (dialog if empty)"=w3820, "2D data"=w3825) -> ()  [unwired: 12 in, 2 out]
          n2665 = Concatenate Strings("StimPresets_" ("name or relative path"), w3810, w3812, w3815, w3814) -> (w3818:string)
          n2666 = Build Path(base path=w3813, name or relative path=w3818) -> (appended path=w3817:path)
          n2667 = call-poly <vilib>:"Write Delimited Spreadsheet.vi"("file path (dialog if empty)"=w3817, "2D data"=w3809) -> ()  [unwired: 12 in, 2 out]
        }
        frame #2 {
          # "Stopping NIP recording and moving unnamed data files into the appropriate data folder on drive D:"
          n2668 = local read "DecodeClust"() -> (w3832:T5)
          n2669 = Bundle By Name(cluster=w3832, "EventStr"="SS.Stop=1;") -> (w3829:T5)
          n2670 = call "FeedbackDecode_MLComCtrl.vi"("DecodeClustIn"=w3829, "Mode"=T19."SendEvent") -> ("DecodeClustOut"=w3828:T5)  [unwired: 6 in, 3 out]
          n2671 = call "FeedbackDecode_MLComCtrl.vi"("DecodeClustIn"=w3828, "Mode"=T19."Wait") -> ("DecodeClustOut"=w3827:T5)  [unwired: 6 in, 3 out]
          n2672 = Bundle By Name(cluster=w3827, "CtrlButtons.Stop"=FALSE) -> (w3826:T5)
          n2673 = local write "DecodeClust"(w3826) -> ()
        }
        frame #3 {
          # "Copy files from RemoteRepo on Matlab computer"
          n2674 = local read "DecodeClust"() -> (w3835:T5)
          n2675 = Unbundle By Name(w3835) -> ("NumComp"=w3836:enum16{"1 Computer", "2 Computers"})
          n2676 = case shown="\"2 Computers\", Default" w3836 {
            tunnel: w3835 -> [_ w3837]
            frame "1 Computer" {
            }
            frame "2 Computers", Default {
              n2677 = call "FeedbackDecode_MLComCtrl.vi"("DecodeClustIn"=w3837, "Mode"=T19."CopyTraining") -> ()  [unwired: 6 in, 4 out]
            }
          }
        }
        frame #4 {
          n2678 = call "Data options"() -> ("Delete from D drive?"=→"Delete from D drive?":bool, "Copy to raid?"=→"Copy to raid?":bool, "Don't save to database?"=→"Don't save to database?":bool)  [unwired: 15 in, 2 out]
        }
        frame #5 {
          # "add to database"
          n2679 = local read "Don't save to database?"() -> (w3842:bool)
          n2680 = case shown="False" w3842 {
            frame False {
              n2681 = local read "DecodeClust"() -> (w3844:T5)
              n2682 = local read "ExperimentDate"() -> (w3850:timestamp)
              n2683 = local read "TaskType"() -> (w3849:string)
              n2684 = Unbundle By Name(w3844) -> ("DataFolder"=w3843:string)
              n2685 = Empty String/Path?(string/path=w3843) -> (empty?=w3845:bool)
              n2686 = local read "Database"() -> (w3851:T12)
              n2687 = Bundle By Name(cluster=w3851, "ExperimentDate"=w3850, "CerebusFolder"=w3843, "TaskType"=w3849) -> (w3846:T12)
              n2688 = case shown="True" w3845 {
                frame False {
                }
                frame True {
                  n2689 = One Button Dialog(message="The data folder is unknown and will not be saved to the database. Make sure to update the database manually with the appropriate folder name!") -> ()  [unwired: 1 in, 1 out]
                }
              }
              n2690 = local read "DatabaseUDL"() -> (w3848:path)
              n2691 = local write "Database"(w3846) -> ()
              n2692 = call "FeedbackDecode_UpdateDatabase.vi"("DatabaseIn"=w3846, "CallType"=enum16{"Initialize", "Save", "Load"}."Save", "DatabaseUDL"=w3848) -> ()  [unwired: 1 in, 3 out]
            }
            frame True {
            }
          }
        }
        frame #6 {
          # "copy to raid"
          n2693 = flat-sequence {
            frame #0 {
              "CopySucc" <- FALSE
            }
            frame #1 {
              n2694 = local read "Copy to raid?"() -> (w3854:bool)
              n2695 = case shown="True" w3854 {
                frame False {
                }
                frame True {
                  n2696 = local read "DecodeClust"() -> (w3859:T5)
                  n2697 = local read "Database"() -> (w3858:T12)
                  n2698 = Unbundle By Name(w3858) -> ("PatientNumber"=w3855:string)
                  n2699 = Unbundle By Name(w3859) -> ("DataFolder"=w3857:string)
                  n2700 = Empty String/Path?(string/path=w3855) -> (empty?=w3856:bool)
                  n2701 = case shown="False" w3856 {
                    tunnel: w3857 -> [w3867 _]
                    tunnel: w3855 -> [w3865 _]
                    frame False {
                      n2702 = Concatenate Strings("E:\\Data\\" ("string"), w3865, "\\" ("string"), w3867) -> (w3868:string)
                      n2703 = String To Path(string=w3868) -> (path=w3860:path)
                      n2704 = Strip Path(path=w3860) -> (stripped path=w3861:path)  [unwired: 1 out]
                      n2705 = call <vilib>:"Check if File or Folder Exists.vi"("path"=w3861) -> ("error out"=w3863:errorcluster, "file or folder exists?"=w3862:bool)  [unwired: 8 in, 1 out]
                      n2706 = case shown="True" w3862 {
                        tunnel: w3863 -> [_ w3872]
                        tunnel: w3860 -> [_ w3873]
                        frame False {
                          n2707 = One Button Dialog(message="Cannot copy to raid. Patient folder does not exist on raid.") -> ()  [unwired: 1 in, 1 out]
                        }
                        frame True {
                          n2708 = local read "DataPath"() -> (w3874:path)
                          n2709 = Copy(8:w3872, 10:w3873, 11:w3874) -> (1:w3871:bool)  [unwired: 2 in, 2 out]
                          n2710 = Not(x=w3871) -> (.not. x?=w3870:bool)
                          n2711 = local write "CopySucc"(w3870) -> ()
                        }
                      }
                    }
                    frame True {
                      n2712 = One Button Dialog(message="Cannot copy to raid. Patient number is missing in database.") -> ()  [unwired: 1 in, 1 out]
                    }
                  }
                }
              }
            }
          }
        }
        frame #7 {
          w3879 = FALSE ("Blinking")
          n2713 = local read "RespRefArray"() -> (w3878:refnum<vi>[])
          n2714 = disable-structure shown="Disabled" {
            frame Disabled {
              n2715 = vi-ref "FeedbackDecode_MSMS2DEKA.vi"() -> (w3893:refnum<vi>)
              n2716 = property class="VI"(reference=w3893) -> (reference out=w3891:refnum<vi>, "FP.State"=w3892:T21)  [unwired: 1 in, 1 out]
              n2717 = case shown="\"Standard\", Default" w3892 {
                tunnel: w3891 -> [_ w3894]
                frame "Closed" {
                }
                frame "Standard", Default {
                  n2718 = invoke class="VI" method="FP.Close"(reference=w3894) -> ()  [unwired: 2 in, 3 out]
                }
              }
            }
            frame Enabled {
            }
          }
          n2719 = for {
            tunnel: w3878 -> [w3895] mode=indexing
            n2720 = property class="VI"(reference=w3895) -> (reference out=w3897:refnum<vi>, "FP.State"=w3896:T21)  [unwired: 1 in, 1 out]
            n2721 = case shown="\"Standard\", Default" w3896 {
              tunnel: w3897 -> [_ w3898]
              frame "Closed" {
              }
              frame "Standard", Default {
                n2722 = invoke class="VI" method="FP.Close"(reference=w3898) -> ()  [unwired: 2 in, 3 out]
              }
            }
          }
          n2723 = disable-structure shown="Disabled" {
            frame Disabled {
              n2724 = vi-ref "FeedbackDecode_AllEMGHM.vi"() -> (w3899:refnum<vi>)
              n2725 = invoke class="VI" method="FP.Close"(reference=w3899) -> ()  [unwired: 2 in, 3 out]
            }
            frame Enabled {
            }
          }
          n2726 = local write "LVTab"(enum32{"Decode", "Encode", "Video", "Database"}."Decode" ("LVTab")) -> ()
          n2727 = local read "EncodeClust"() -> (w3881:T9)
          n2728 = local read "DecodeClust"() -> (w3884:T5)
          n2729 = local read "EventParamsFID"() -> (w3885:refnum<file>)
          n2730 = local read "PSRef"() -> (w3889:refnum<vi>)
          n2731 = Close Reference(reference=w3889) -> ()  [unwired: 1 in, 1 out]
          n2732 = call "FeedbackDecode_MLComCtrl.vi"("DecodeClustIn"=w3884, "EncodeClustIn"=w3881, "Mode"=T19."Close") -> ("DecodeClustOut"=w3883:T5, "EncodeClustOut"=w3882:T9)  [unwired: 5 in, 2 out]
          n2733 = call "FeedbackDecode_SendMSMSPacket.vi"("Mode"=enum16{"Initialize", "Run", "Close"}."Close") -> ()  [unwired: 6 in]
          n2734 = Close File(refnum=w3885) -> ()  [unwired: 1 in, 2 out]
          n2735 = local write "EncodeClust"(w3882) -> ()
          n2736 = local write "DecodeClust"(w3883) -> ()
          n2737 = local read "DAQmx?"() -> (w3876:bool)
          n2738 = case shown="True" w3876 {
            frame False {
            }
            frame True {
              n2739 = call <vilib>:"DAQmx Stop Task.vi"("task/channels in"=refnum<k21> "AO0") -> ()  [unwired: 13 in, 2 out]
            }
          }
          n2740 = global write "FeedbackDecode_Globals.vi" "FD_Stop"(FALSE ("G_Stop")) -> ()
          n2741 = property on="Finished" class="Bool (strict)"("DisabledEnum"=T17."Disabled and Grayed Out" ("Disabled"), "Blinking"=w3879, "Value"=w3879) -> ()  [unwired: 2 in, 2 out]
        }
        frame #8 {
          n2742 = local read "Delete from D drive?"() -> (w3900:bool)
          n2743 = case shown="True" w3900 {
            frame False {
            }
            frame True {
              n2744 = local read "CopySucc"() -> (w3901:bool)
              n2745 = case shown="False" w3901 {
                frame False {
                  n2746 = Two Button Dialog(message="Data was not copied to raid. Delete anyway? ", 2:"Yes" ("T button name (\"OK\")")) -> (T button?=w3902:bool)  [unwired: 1 in]
                  n2747 = case shown="True" w3902 {
                    frame False {
                    }
                    frame True {
                      w3905 = TRUE ("confirm (F)")
                      n2748 = local read "DataPath"() -> (w3906:path)
                      n2749 = Delete(path (use dialog)=w3906, entire hierarchy (F)=w3905, confirm (F)=w3905) -> ()  [unwired: 2 in, 3 out]
                    }
                  }
                }
                frame True {
                  w3907 = TRUE ("confirm (F)")
                  n2750 = local read "DataPath"() -> (w3908:path)
                  n2751 = Delete(path (use dialog)=w3908, entire hierarchy (F)=w3907, confirm (F)=w3907) -> ()  [unwired: 2 in, 3 out]
                }
              }
            }
          }
        }
      }
    }
  }
